vi "Delete from DataBase.vi"(8 "error in (no error)":errorcluster, 10 "Item ID":string, 11 "Customer DAO JSON in":refnum<class "Object DAO JSON.lvclass">) -> (0 "error out":errorcluster, 3 "Customer DAO JSON out":refnum<class "Object DAO JSON.lvclass">)   [LabVIEW 2020, in "Object DAO JSON.lvclass"]
uses:
  Object DAO JSON.lvclass
  Object DAO JSON.lvclass/Object DAO JSON.ctl
  <vilib>/JDP Science/JSONtext/JSONtext.lvlib
  External Libraries/JSON File Manipulation.lvlibp
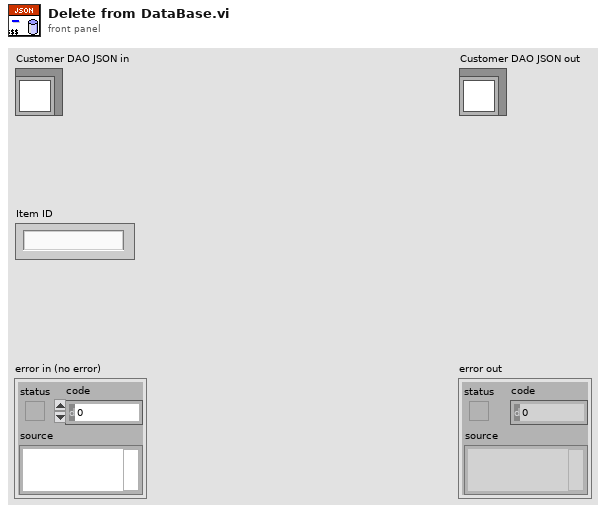
[diagram p1: front panel]
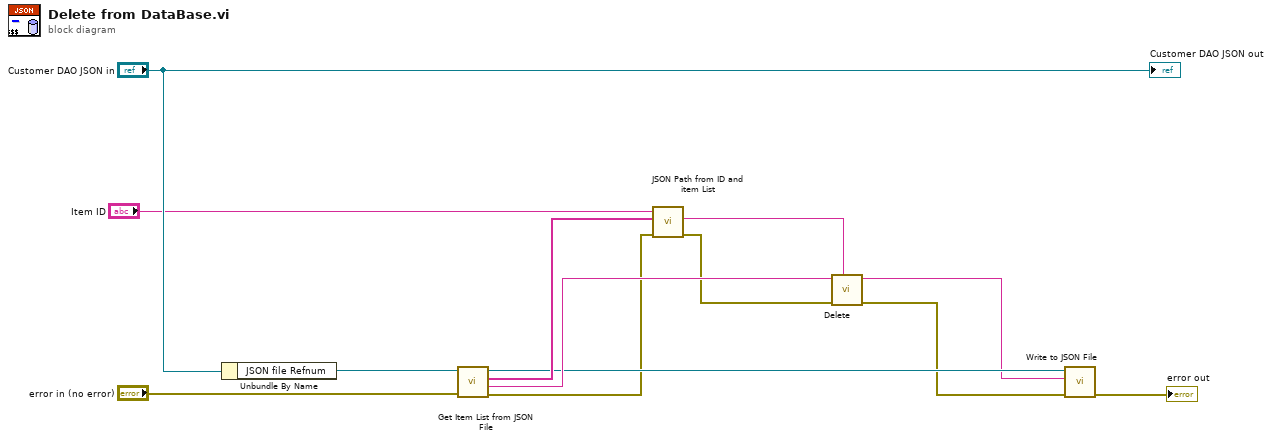
[diagram p0: block diagram]
diagram:
  n1 = Unbundle By Name("Customer DAO JSON in") -> ("JSON file Refnum"=w10:refnum<file>)
  n2 = call "Get Item List from JSON File.vi"("error in (no error)"="error in (no error)", "Byte Stream File in"=w10) -> ("error out"=w1:errorcluster, "JSON String"=w12:string, "Item List"=w13:string[], "Byte Stream File out"=w11:refnum<file>)  [unwired: 6 in]
  n3 = call "JSON Path from ID and item List.vi"("error in (no error)"=w1, "Item List"=w13, "Item ID"="Item ID") -> ("error out"=w2:errorcluster, "Item JSON string"=w4:string)  [unwired: 7 in]
  n4 = call <vilib>:"Delete.vi"("$Path or Item Name"=w4, "error in (no error)"=w2, "JSON"=w12) -> ("error out"=w3:errorcluster, "<JSON>"=w5:string)  [unwired: 4 in, 2 out]
  n5 = call "Write to JSON File.vi"("error in (no error)"=w3, "JSON String"=w5, "Byte Stream File in"=w11) -> ("error out"=→"error out":errorcluster)  [unwired: 8 in]
  "Customer DAO JSON out" <- "Customer DAO JSON in"
